vi "Main.vi"() -> ()   [LabVIEW 2020, in "MacroAssert.lvlib" / "Win Util.lvlib"]
uses:
  Win Util.lvlib
  d12568f4-0a9c-4951-98c0-f994682667d9.vi
panel:
  in  "Key Delay":u32=5
  out "Equal?":bool
  in  "Recreate":bool
  in  "Stop Button":bool
  out "error out":errorcluster
  in  "Update Here":string
  in  "String Input":string
  in  "error in (no error)":errorcluster
  # "Overview: Demonstrates the use of VkKeyScanExA() to convert a string to virtual keys and use of SendInput() to synthesise that string being typed.\nRequirements: LabVIEW  2016 Base Development System\nInstructions:\n1) Run the VI.\n2) Type a string into the String Input field.\n3) Click the \"Recreate String\" Button."
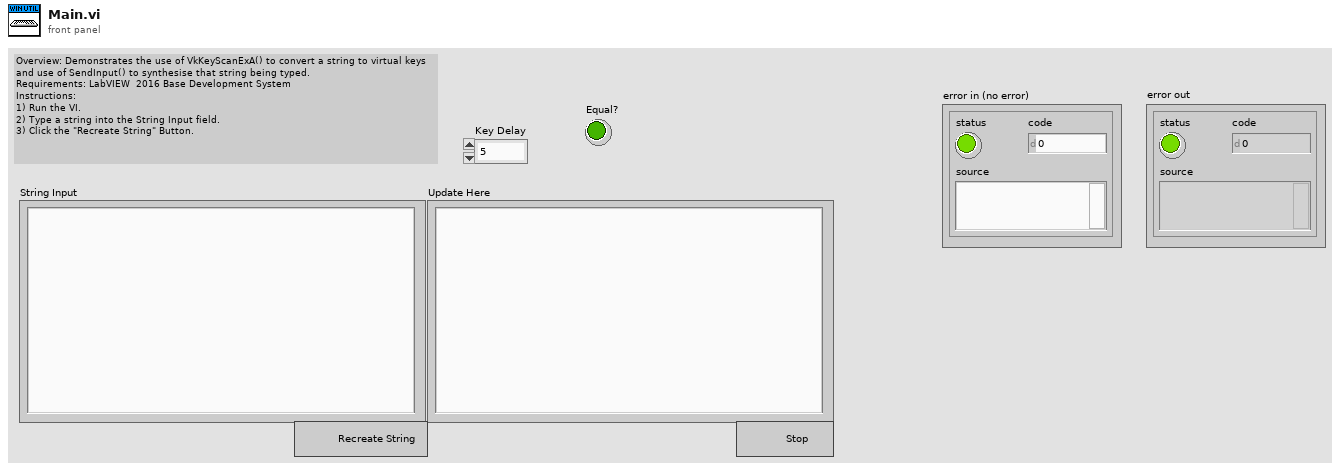
[diagram p1: front panel]
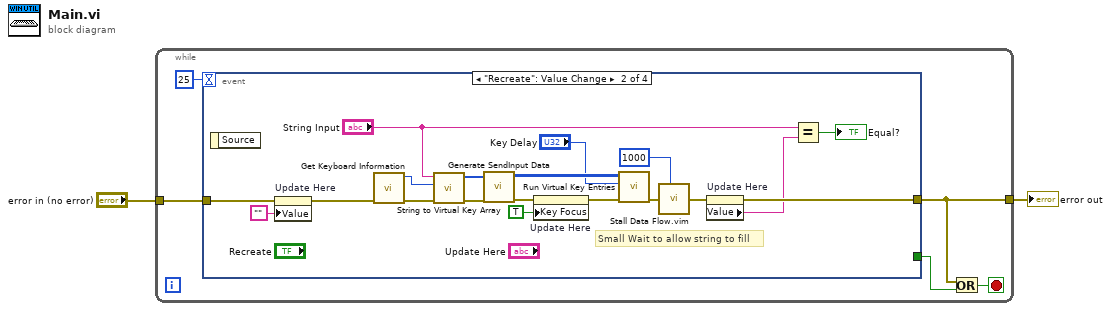
[diagram p0: block diagram]
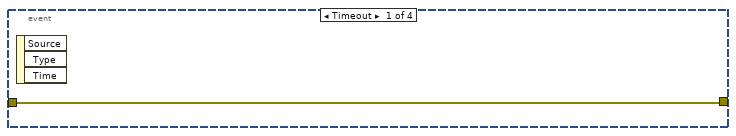
[diagram p2: hidden frame]
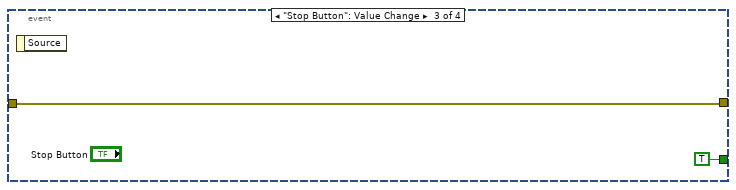
[diagram p3: hidden frame]
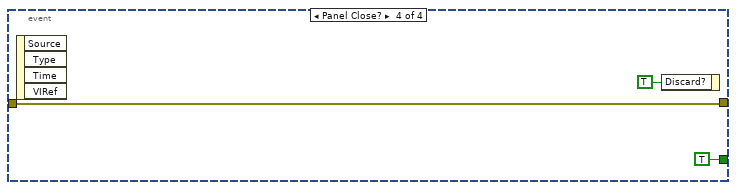
[diagram p4: hidden frame]
diagram:
  n1 = while {
    tunnel: "error in (no error)" -> [w6]
    tunnel: [w3] -> w1
    stop <- w4 stop-if-true
    n2 = event shown="[1] \"Recreate\": Value Change" {
      selector: _ -> [_ _ _ _]
      dyn-events: _ -> [_ _ _ _]
      timeout: 25 -> [_ _ _ _]
      tunnel: [w8 w15 w28 w31] -> w3
      tunnel: w6 -> [w8 w17 w28 w31]
      tunnel: [_ _ TRUE TRUE] -> w5
      event Timeout {
        n3 = event-data() -> ()  [unwired: 1 in, 3 out]
      }
      event "Recreate": Value Change {
        # "Small Wait to allow string to fill"
        n4 = event-data() -> ()  [unwired: 1 in, 1 out]
        n5 = property on="Update Here" class="Str"(error in=w17, "Value"="") -> (error out=w27:errorcluster)  [unwired: 1 in, 1 out]
        n6 = call "Get Keyboard Information.vi"("error in (no error)"=w27) -> ("error out"=w19:errorcluster, "HKL"=w18:u64)  [unwired: 9 in]
        n7 = call "String to Virtual Key Array.vi"("error in (no error)"=w19, "Keyboard Type"=w18, "String"="String Input") -> ("error out"=w21:errorcluster, "Array"=w20:u16[])  [unwired: 7 in]
        n8 = call "Generate SendInput Data.vi"("error in (no error)"=w21, "Array"=w20) -> ("error out"=w23:errorcluster, "Key Press Array"=w22:u8[][])  [unwired: 8 in]
        n9 = property on="Update Here" class="Str"(error in=w23, "Key Focus"=TRUE) -> (error out=w24:errorcluster)  [unwired: 1 in, 1 out]
        n10 = call "Run Virtual Key Entries.vi"("error in (no error)"=w24, "Key Delay"="Key Delay", "Key Press Array"=w22) -> ("error out"=w16:errorcluster)  [unwired: 8 in]
        n11 = call "Stall Data Flow.vim"("value in"=w16, "milliseconds to wait"=u32 1000) -> ("value out"=w11:errorcluster)  [unwired: 1 out]
        n12 = property on="Update Here" class="Str"(error in=w11) -> (error out=w15:errorcluster, "Value"=w14:string)  [unwired: 1 in, 1 out]
        n13 = Equal?(x="String Input", y=w14) -> (x = y?=→"Equal?":bool)
      }
      event "Stop Button": Value Change {
        n14 = event-data() -> ()  [unwired: 1 in, 1 out]
      }
      event Panel Close? {
        n15 = event-data() -> ()  [unwired: 1 in, 4 out]
        n16 = event-data("Discard?"=TRUE) -> ()  [unwired: 1 in, 1 out]
      }
    }
    n17 = Or(x=w3, y=w5) -> (x .or. y?=w4:bool)
  }
  "error out" <- w1
